vi "mostCommonValue.vi"(11 "Array":i32[](array[numeric])) -> (2 "Minor":i32, 3 "Major":i32)   [LabVIEW 2017]
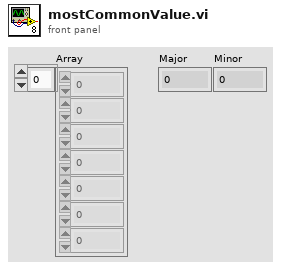
[diagram p1: front panel]
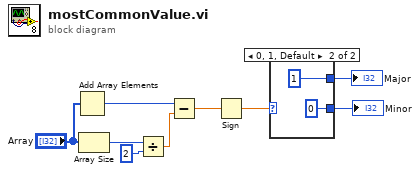
[diagram p0: block diagram]
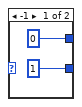
[diagram p2: hidden frame]
diagram:
  n1 = Add Array Elements(numeric array="Array") -> (sum=w8:i32)
  n2 = Array Size(array="Array") -> (size(s)=w4:i32)
  n3 = Divide(x=w4, y=2) -> (x/y=w2:dbl)
  n4 = Subtract(x=w8, y=w2) -> (x-y=w7:dbl)
  n5 = Sign(1:w7) -> (0:w6:dbl)
  n6 = case shown="0, 1, Default" w6 {
    tunnel: [0 1] -> w5
    tunnel: [1 0] -> w1
    frame -1 {
    }
    frame 0, 1, Default {
    }
  }
  "Major" <- w5
  "Minor" <- w1
